vi "Stop Driving.vi"(1 "Execute":bool) -> (4 "Done Executing":bool)   [LabVIEW 2012]
uses:
  Globals/Autonomous Joystick Emulation.vi
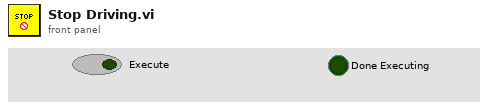
[diagram p1: front panel]
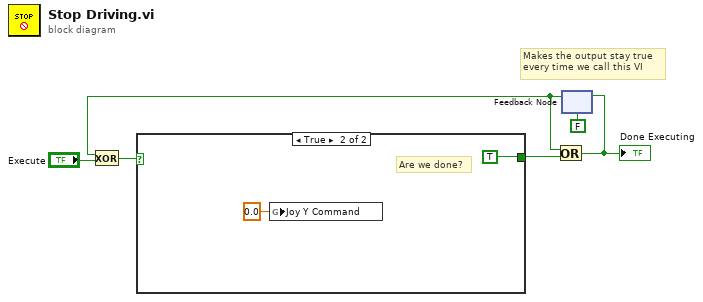
[diagram p0: block diagram]
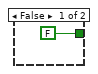
[diagram p2: hidden frame]
diagram:
  # "Makes the output stay true\nevery time we call this VI"
  n1 = feedback #1(FALSE) -> (w2:bool)
  n2 = Exclusive Or(1:"Execute", 2:w2) -> (0:w6:bool)
  n3 = case shown="True" w6 {
    tunnel: [FALSE TRUE] -> w4
    frame False {
    }
    frame True {
      # "Are we done?"
      n4 = global write "Autonomous Joystick Emulation.vi" "Joy Y Command"(0.0 ("Joy Y Command")) -> ()
    }
  }
  n5 = Or(x=w2, y=w4) -> (x .or. y?=w1:bool)
  "Done Executing" <- w1
  n6 = feedback-in #1(w1) -> ()
